vi "editDialog.vi"(0 "reference":refnum<class "ClassRelationshipEdge.lvclass">, 5 "error in (no error)":errorcluster) -> (14 "reference out":refnum<class "ClassRelationshipEdge.lvclass">, 15 "cancel":bool, 19 "error out":errorcluster)   [LabVIEW 2016, in "ClassRelationshipEdge.lvclass"]
doc: "Edit Dialog"
uses:
  <resource>/Framework/Providers/Open_GDS/UML/ClassRelationshipEdge_class/ClassRelationshipEdge.lvclass
  <resource>/Framework/Providers/Open_GDS/UML/ArrowHead_class/ArrowHeadType.ctl
  C:/Program Files (x86)/National Instruments/LabVIEW 2016/resource/Framework/Providers/Open_GDS/UML/SegmentedLineEdge_class/SegmentedLineEdge.lvclass
  <resource>/Framework/Providers/Open_GDS/UML/ContextHelp/ContextHelp_HelpTexts.ctl
  <resource>/Framework/Providers/Open_GDS/UML/ClassRelationshipEdge_class/private/AssociationType.ctl
  <resource>/Framework/Providers/Open_GDS/UML/BentStyle_class/BentStyle.lvclass
  <resource>/Framework/Providers/Open_GDS/UML/LineStyle_class/LineStyle.lvclass
  <resource>/Framework/Providers/Open_GDS/UML/ArrowHead_class/ArrowHead.lvclass
  <resource>/Framework/Providers/Open_GDS/UML/SegmentedLineEdge_class/SegmentedLineEdge.lvclass
panel:
  in  "SplitWire":bool
  in  "Bent Style 2":enum16{"STRAIGHT", "HV", "VH", "HVH", "VHV"}(ring) caption="bentStyle"
  in  "Help":bool
  in  "Bi directional":bool
  in  "Reverse association":bool
  in  "RelationType":u16(ring) items=["Dependency", "Inheritance", "Interface Implementation", "Association", "Aggregation", "Composite Aggregation"]
  in  "Line style":enum16{"SOLID", "DOTTED"}(ring)
  in  "Middle label":string(combo)
  in  "Start arrow head":T1
  in  "End arrow head":T1
  in  "Bent Style":enum16{"STRAIGHT", "HV", "VH", "HVH", "VHV"}(ring) caption="bentStyle"
  in  "Start label":string
  in  "End label":string
  in  "Cancel Button":bool
  in  "OK Button":bool
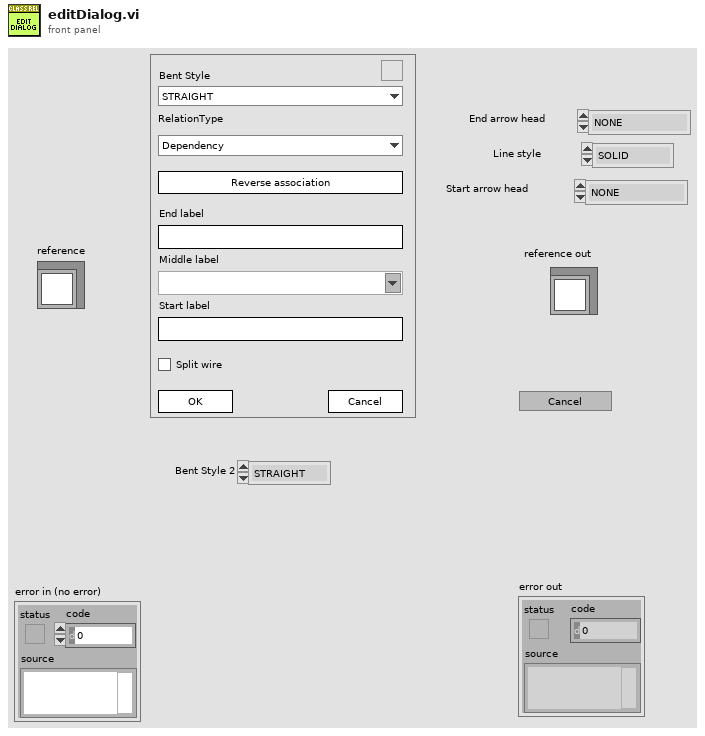
[diagram p1: front panel]
types:
  T1 = typedef "ArrowHead.lvclass/ArrowHeadType.ctl" = enum16{"NONE", "TRIANGLE", "BLACK_TRIANGLE", "V", "HALF_V", "DIAMOND", "BLACK_DIAMOND"}
  T2 = typedef "ContextHelp_HelpTexts.ctl" = enum16{"None(Hide)", "Default", "Help", "Welcome", "GettingStarted", "ClassDiagram_Help", "SequenceDiagram_Help", "UseCaseDiagram_Help", "BSelect", "BClass", "BInterface", "BPackage", "BNote", "BDependency", "BInheritance", "BInterfaceImplementation", "BAssociation", "BAggregation", "BCompAggregation", "BNoteConnector", "BObject", "BActionBar", "BCall", "BSystem", "BActor", "BUseCase", "BGeneralization", "BIncludes", "BExtends", "BUseCaseDiagramAssociation", "ClassRelationshipEdge editDialog_Bent Style", "ClassRelationshipEdge editDialog_RelationType", "ClassRelationshipEdge editDialog_Reverse association", "ClassRelationshipEdge editDialog_Start label", "ClassRelationshipEdge editDialog_Middle label", "ClassRelationshipEdge editDialog_End label", "UMLEditor reversedEngineering_Pathes", "ReversedEngineering StateReverseDialog_Help", "ReversedEngineering StateQueuedSettings_Help", "UMLEditor reversedEngineering_AddTopVIs", "UMLEditor reversedEngineering_AddClasses", "UMLEditor reversedEngineering_AddDirs", "UMLEditor reversedEngineering_Recursively", "UMLEditor reversedEngineering_Remove", "UMLEditor reversedEngineering_ClearList", "UMLEditor reversedEngineering_HideSubAss", "UMLEditor reversedEngineering_CreateTypes", "UMLEditor reversedEngineering_OnlyInheritance", "UMLEditor reversedEngineering_CreateApplication", "UMLEditor reversedEngineering_OK", "UMLEditor reversedEngineering_Cancel", "UMLEditor reversedEngineering_Help", "UMLEditor createWizardScriptFile_ScriptfilePath", "UMLEditor createWizardScriptFile_ClassPath", "UMLEditor createWizardScriptFile_Use", "UMLEditor createWizardScriptFile_PrivateDirName", "UMLEditor createWizardScriptFile_DirAppend", "UMLEditor createWizardScriptFile_Separator Character", "UMLEditor createWizardScriptFile_OK", "UMLEditor createWizardScriptFile_Cancel", "UMLEditor createWizardScriptFile_Help", "ClassNode editDialog_Class Name", "InterfaceNode editDialog_Class Name", "ClassNode editDialog_Attribute", "ClassNode editDialog_Methods", "InterfaceNode editDialog_Methods", "ClassNode editDialog_connection", "InterfaceNode editDialog_connection", "ClassNode editDialog_StereoType", "ClassNode editDialog_ShowAttrib", "ClassNode editDialog_ShowMethods", "ClassNode editDialog_ClassPath", "ClassNode editDialog_AddAttribute", "ClassNode editDialog_AddMethod", "InterfaceNode editDialog_AddMethod", "ClassNode AttributeGuide_AttributeName", "ClassNode AttributeGuide_Array?", "ClassNode AttributeGuide_Data Type", "ClassNode AttributeGuide_RefName", "ClassNode AttributeGuide_Preview", "ClassNode AttributeGuide_OK", "ClassNode AttributeGuide_Cancel", "ClassNode MethodGuide_Visibility", "ClassNode MethodGuide_Method Name", "ClassNode MethodGuide_Preview", "ClassNode MethodGuide_OK", "ClassNode MethodGuide_Cancel", "CallNode EditCallProperties_AllButtons", "ObjectNode EditObjectlProperties_AllButtons", "ActorNode EditActorProperties_AllButtons", "UseCaseRelationshipNode EditUseCaselProperties_AllButtons", "UseCaseNode EditUseCaselProperties_AllButtons", "SystemNode EditSystemProperties_AllButtons", "ReversedEngineering UpdateAttributes_AllButtons", "StateNode editDialog_AllButtons", "StateTransition editDialog_AllButtons", "ArrangeNodes Main_Picture", "ArrangeNodes Main_Zoom", "ArrangeNodes Main_Auto Zoom", "ArrangeNodes Main_shorten", "ArrangeNodes Main_Min Length", "ArrangeNodes Main_Max Length", "ArrangeNodes Main_increase", "ArrangeNodes Main_decrease", "ArrangeNodes Main_Shake", "ArrangeNodes Main", "BState", "BInitialState", "BFinalState", "BStateTransition", "StateDiagram_Help", "StateDiagram_PropertiesAllButtons", "ReversedEngineering StateReverseDialog_ClearStates", "ReversedEngineering StateReverseDialog_UseQueuedStateMachines", "ReversedEngineering StateReverseDialog_QueuedSettings", "ReversedEngineering StateReverseDialog_SearchForVIs", "ReversedEngineering StateReverseDialog_SearchCriteria", "OptionsDialog_ClassBasePath", "OptionsDialog_VIPath", "OptionsDialog_ApplicationPath", "OptionsDialog_WizDir", "OptionsDialog_IniFilePath", "OptionsDialog_DefineColors", "OptionsDialog_Help", "OptionsDialog_CreateTypes", "ClassRelationshipEdge editDialog_SplitWire"}
  T3 = typedef "ClassRelationshipEdge.lvclass/ObjectAttributes.ctl" = cluster{"bentStyleRef":refnum<class "BentStyle.lvclass">, "startConnectionOffset":cluster{"x":i32, "y":i32}, "endConnectionOffset":cluster{"x":i32, "y":i32}, "MidLineOffset":cluster{"x":i32, "y":i32}, "DepClass":T4}
  T4 = typedef "ReversedEngineering_ViDependencyDetailsType.ctl" = cluster{"ThisVIs/Ctls":path[], "Dependent_VIs/Ctls":path[]}
  T5 = typedef "SegmentedLineEdge.lvclass/ObjectAttributes.ctl" = cluster{"lineStyle":refnum<class "LineStyle.lvclass">, "startArrowHead":refnum<class "ArrowHead.lvclass">, "endArrowHead":refnum<class "ArrowHead.lvclass">, "startLabel":string, "midLabel":string, "endLabel":string, "MidLabelOffset":T6, "SplitWire":bool}
  T6 = typedef "Point Point2D.ctl" = cluster{"x":dbl, "y":dbl}
  T7 = typedef "ContextHelp_ShowType.ctl" = cluster{"Header":string, "Picture":picture, "Text":string}
  T8 = typedef "ClassRelationshipEdge.lvclass/AssociationType.ctl" = u16
  T9 = typedef "BentStyle.lvclass/BentStyleType.ctl" = enum16{"STRAIGHT", "HV", "VH", "HVH", "VHV", "ARC"}
  T10 = typedef "LineStyle.lvclass/LineStyleType.ctl" = enum16{"SOLID", "DOTTED"}
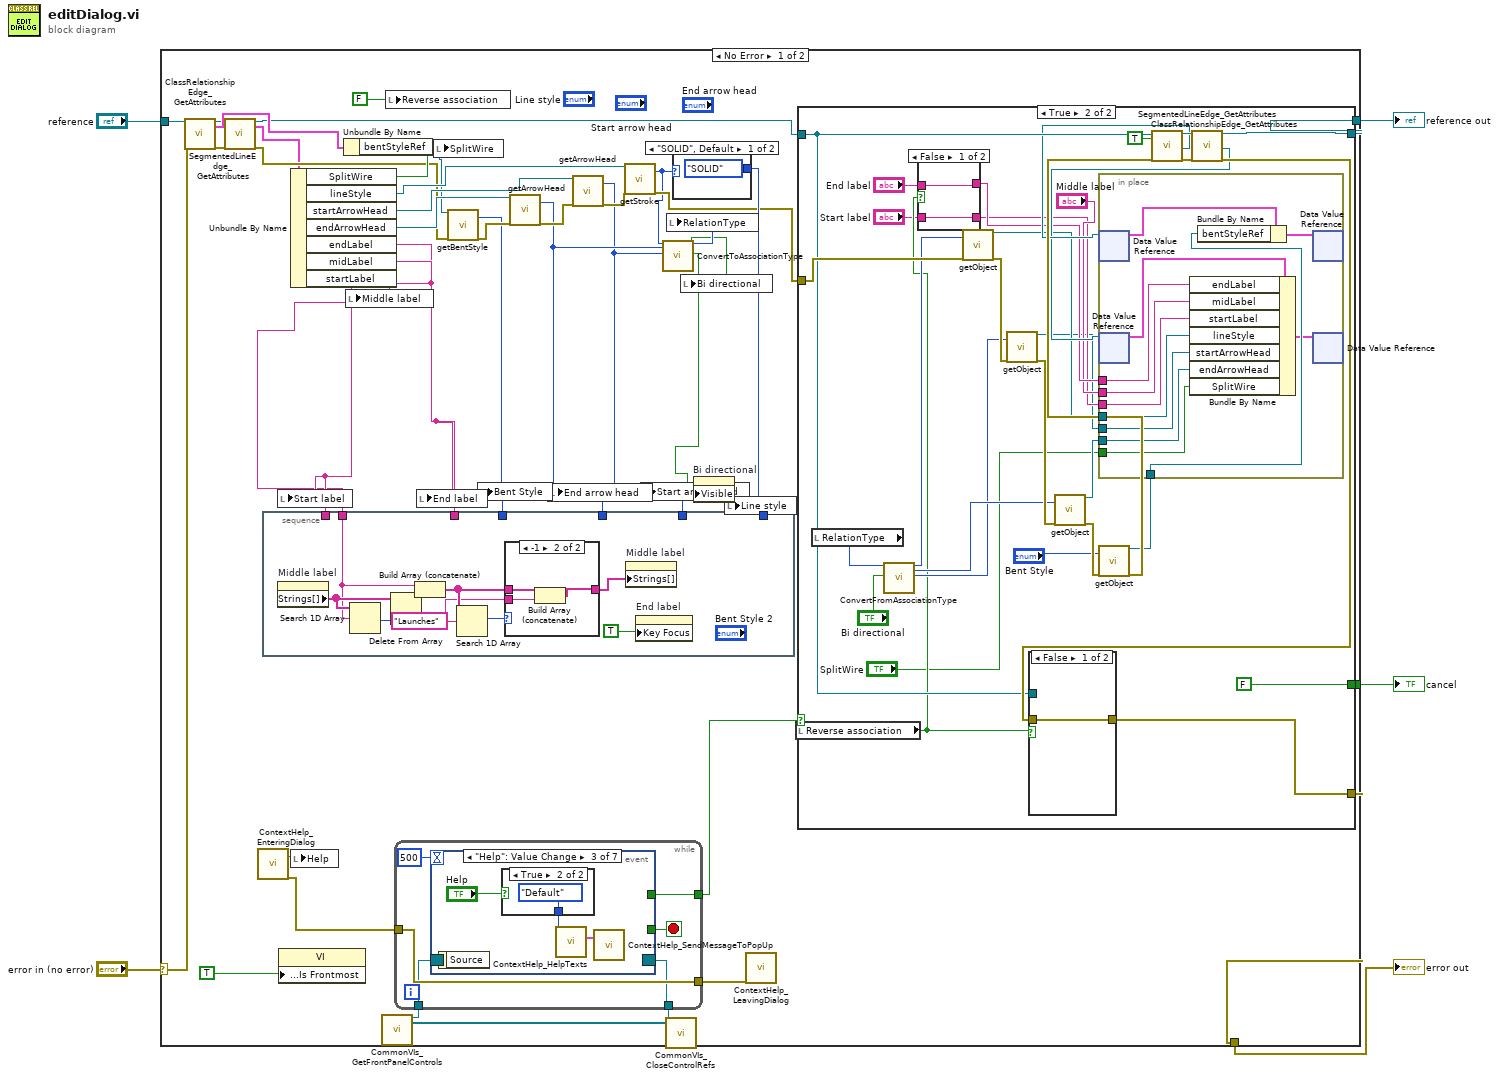
[diagram p0: block diagram]
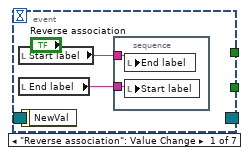
[diagram p2: hidden frame]
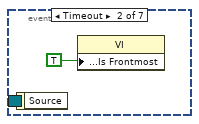
[diagram p3: hidden frame]
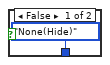
[diagram p4: hidden frame]
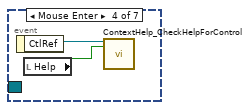
[diagram p5: hidden frame]
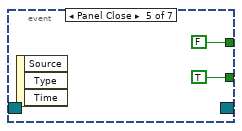
[diagram p6: hidden frame]
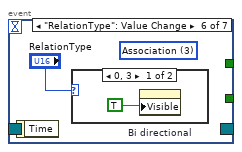
[diagram p7: hidden frame]
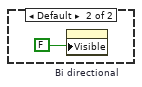
[diagram p8: hidden frame]
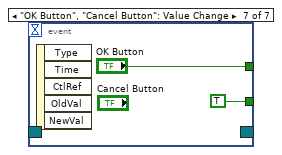
[diagram p9: hidden frame]
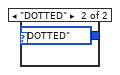
[diagram p10: hidden frame]
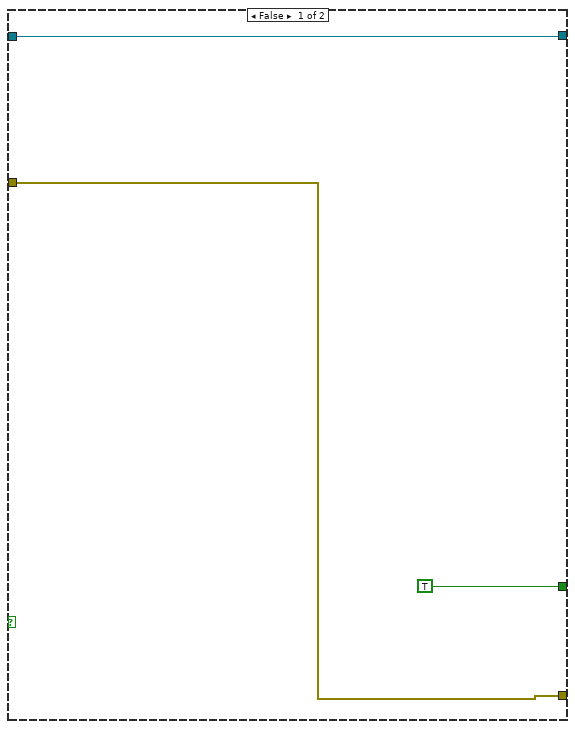
[diagram p11: hidden frame]
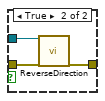
[diagram p13: hidden frame]
diagram:
  n1 = case shown="No Error" "error in (no error)" {
    selector: "error in (no error)" -> [w41 w140]
    tunnel: "reference" -> [w42 w141]
    tunnel: [w44 w140] -> w3
    tunnel: [w43 w141] -> w2
    tunnel: [w26 _] -> w1
    frame No Error {
      n2 = call <resource>:"ClassRelationshipEdge_GetAttributes.vi"("reference in"=w42, "error in (no error)"=w41) -> ("reference out"=w10:refnum<class "ClassRelationshipEdge.lvclass">, "Data"=w11:T3, "error out"=w9:errorcluster)  [unwired: 1 in, 14 out]
      n3 = call <resource>:"SegmentedLineEdge_GetAttributes.vi"("reference in"=w10, "error in (no error)"=w9) -> ("reference out"=w7:refnum<class "ClassRelationshipEdge.lvclass">, "Data"=w6:T5, "error out"=w8:errorcluster)  [unwired: 14 in, 1 out]
      n4 = call <resource>:"ContextHelp_EnteringDialog.vi"() -> ("HelpStatus"=w19:bool, "error out"=w18:errorcluster)  [unwired: 3 in, 15 out]
      n5 = property class="VI"("Front Panel Window:Is Frontmost"=TRUE) -> ()  [unwired: 2 in, 2 out]
      n6 = Unbundle By Name(w6) -> ("SplitWire"=w12:bool, "lineStyle"=w39:refnum<class "LineStyle.lvclass">, "startArrowHead"=w35:refnum<class "ArrowHead.lvclass">, "endArrowHead"=w33:refnum<class "ArrowHead.lvclass">, "endLabel"=w36:string, "midLabel"=w37:string, "startLabel"=w38:string)
      n7 = local write "Start label"(w38) -> ()
      n8 = local write "Help"(w19) -> ()
      n9 = Unbundle By Name(w11) -> ("bentStyleRef"=w30:refnum<class "BentStyle.lvclass">)
      n10 = local write "Middle label"(w37) -> ()
      n11 = call <resource>:"CommonVIs_GetFrontPanelControls.vi"() -> ("Event Registration Refnum"=w15:refnum<event-registration>, "ControlRefs"=w13:refnum<vi>[])  [unwired: 2 in, 16 out]
      n12 = local write "Reverse association"(FALSE ("Reverse association")) -> ()
      n13 = while {
        tunnel: [w50] -> w40
        tunnel: w18 -> [w48]
        tunnel: [w48] -> w17
        tunnel: w15 -> [w46]
        tunnel: [w45] -> w14
        stop <- w49 stop-if-true
        n14 = event shown="[2] \"Help\": Value Change" {
          selector: w46 -> [_ _ _ _ _ _ _]
          dyn-events: [_ _ _ _ _ _ _] -> w45
          timeout: 500 -> [_ _ _ _ _ _ _]
          tunnel: [_ _ _ _ FALSE ("OK Button") _ "OK Button"] -> w50
          tunnel: [_ _ _ _ TRUE _ TRUE] -> w49
          event "Reverse association": Value Change {
            n15 = local read "Start label"() -> (w52:string)
            n16 = local read "End label"() -> (w51:string)
            n17 = event-data() -> ()  [unwired: 2 out]
            n18 = stacked-sequence {
              tunnel: w52 -> [w54]
              tunnel: w51 -> [w53]
              frame #0 {
                n19 = local write "End label"(w54) -> ()
                n20 = local write "Start label"(w53) -> ()
              }
            }
          }
          event Timeout {
            n21 = event-data() -> ()  [unwired: 2 out]
            n22 = property class="VI"("Front Panel Window:Is Frontmost"=TRUE) -> ()  [unwired: 2 in, 2 out]
          }
          event "Help": Value Change {
            n23 = event-data() -> ()  [unwired: 2 out]
            n24 = case shown="True" "Help" {
              tunnel: [ContextHelp_HelpTexts."None(Hide)" ("HelpText") ContextHelp_HelpTexts."Default" ("HelpText")] -> w57
              frame False {
              }
              frame True {
              }
            }
            n25 = call <resource>:"ContextHelp_HelpTexts.vi"("HelpText (enum or string)"=w57) -> ("HelpOut"=w58:T7)  [unwired: 18 out]
            n26 = call <resource>:"ContextHelp_SendMessageToPopUp.vi"("PopUpMessage"=w58) -> ()  [unwired: 2 in, 17 out]
          }
          event Mouse Enter {
            n27 = event-data() -> ("CtlRef"=w62:refnum<vi>)  [unwired: 1 out]
            n28 = local read "Help"() -> (w61:bool)
            n29 = call <resource>:"ContextHelp_CheckHelpForControl.vi"("Ctl Refnum"=w62, "Help"=w61) -> ()  [unwired: 1 in, 17 out]
          }
          event Panel Close {
            n30 = event-data() -> ()  [unwired: 4 out]
          }
          event "RelationType": Value Change {
            (unwired) T8 3 items=["Depenency", "Inheritance", "Interface Implementation", "Association", "Aggregation", "Composite Aggregation"] ("RelationType")
            n31 = event-data() -> ()  [unwired: 2 out]
            n32 = case shown="0, 3" "RelationType" {
              frame 0, 3 {
                n33 = property on="Bi directional" class="Bool (strict)"("Visible"=TRUE) -> ()  [unwired: 2 in, 2 out]
              }
              frame Default {
                n34 = property on="Bi directional" class="Bool (strict)"("Visible"=FALSE) -> ()  [unwired: 2 in, 2 out]
              }
            }
          }
          event "OK Button", "Cancel Button": Value Change {
            n35 = event-data() -> ()  [unwired: 6 out]
          }
        }
      }
      n36 = local write "End label"(w36) -> ()
      n37 = local write "SplitWire"(w12) -> ()
      n38 = call-dynamic "getBentStyle.vi"("reference"=w30, "error in (no error)"=w8) -> ("bentStyle"=w27:T9, "error out"=w29:errorcluster)  [unwired: 15 in, 1 out]
      n39 = local write "Bent Style"(w27) -> ()
      n40 = call <resource>:"getArrowHead.vi"("reference"=w33, "error in (no error)"=w29) -> ("arrowHead"=w24:T1, "error out"=w32:errorcluster)  [unwired: 16 out]
      n41 = local write "End arrow head"(w24) -> ()
      n42 = call <resource>:"getArrowHead.vi"("reference"=w35, "error in (no error)"=w32) -> ("arrowHead"=w23:T1, "error out"=w31:errorcluster)  [unwired: 16 out]
      n43 = call-dynamic "getStroke.vi"("reference"=w39, "error in (no error)"=w31) -> ("lineStyle"=w25:T10, "error out"=w28:errorcluster)  [unwired: 15 in, 1 out]
      n44 = local write "Start arrow head"(w23) -> ()
      n45 = call <resource>:"ConvertToAssociationType.vi"("lineStyle"=w25, "EndArrowHead"=w24, "StartArrowHead"=w23) -> ("RelationType"=w22:T8, "Bi sirectional"=w21:bool)  [unwired: 15 out]
      n46 = call <resource>:"CommonVIs_CloseControlRefs.vi"("Event Registration Refnum"=w14, "ControlRefs"=w13) -> ()  [unwired: 1 in, 17 out]
      n47 = local write "RelationType"(w22) -> ()
      n48 = case shown="\"SOLID\", Default" w25 {
        tunnel: [enum16{"SOLID", "DOTTED"}."SOLID" ("Line style") enum16{"SOLID", "DOTTED"}."DOTTED" ("Line style")] -> w34
        frame "SOLID", Default {
        }
        frame "DOTTED" {
        }
      }
      n49 = stacked-sequence {
        tunnel: w34 -> [_]
        tunnel: w38 -> [_]
        tunnel: w37 -> [w132]
        tunnel: w36 -> [_]
        tunnel: w23 -> [_]
        tunnel: w24 -> [_]
        tunnel: w27 -> [_]
        frame #0 {
          w127 = "Launches" ("element")
          n50 = property on="Middle label" class="CmbBox"() -> ("Strings[]"=w134:string[])  [unwired: 2 in, 2 out]
          n51 = Search 1D Array(1D array=w134, element=w132) -> (index of element=w133:i32)  [unwired: 1 in]
          n52 = Delete From Array(array=w134, index=w133) -> (array with subset deleted=w131:string[])  [unwired: 1 in, 1 out]
          n53 = Build Array (concatenate)(w132, w131) -> (w129:string[])
          n54 = Search 1D Array(1D array=w129, element=w127) -> (index of element=w130:i32)  [unwired: 1 in]
          n55 = case shown="-1" w130 {
            tunnel: w129 -> [w136 w139]
            tunnel: [w136 w137] -> w128
            tunnel: w127 -> [_ w138]
            frame 0, Default {
            }
            frame -1 {
              n56 = Build Array (concatenate)(w139, w138) -> (w137:string[])
            }
          }
          n57 = property on="Middle label" class="CmbBox"("Strings[]"=w128) -> ()  [unwired: 2 in, 2 out]
          n58 = property on="End label" class="Str"("Key Focus"=TRUE) -> ()  [unwired: 2 in, 2 out]
        }
      }
      n59 = local write "Bi directional"(w21) -> ()
      n60 = property on="Bi directional" class="Bool (strict)"("Visible"=w21) -> ()  [unwired: 2 in, 2 out]
      n61 = local write "Line style"(w34) -> ()
      n62 = call <resource>:"ContextHelp_LeavingDialog.vi"("error in (no error)"=w17) -> ()  [unwired: 2 in, 17 out]
      n63 = case shown="True" w40 {
        tunnel: [w73 w93] -> w44
        tunnel: [w74 w106] -> w43
        tunnel: w7 -> [w74 w91]
        tunnel: w28 -> [w73 w101]
        tunnel: [TRUE ("Key Focus") FALSE ("Key Focus")] -> w26
        frame False {
        }
        frame True {
          n64 = local read "Reverse association"() -> (w90:bool)
          n65 = local read "RelationType"() -> (w97:u16)
          n66 = call <resource>:"ConvertFromAssociationType.vi"("RelationType"=w97, "Bi sirectional"="Bi directional") -> ("lineStyle"=w98:T10, "EndArrowHead"=w96:T1, "StartArrowHead"=w95:T1)  [unwired: 15 out]
          n67 = case shown="False" w90 {
            tunnel: "End label" -> [w120 w122]
            tunnel: [w119 w122] -> w79
            tunnel: [w120 w121] -> w81
            tunnel: "Start label" -> [w119 w121]
            frame False {
            }
            frame True {
            }
          }
          n68 = call <resource>:"getObject.vi"("lineStyle"=w98, "error in (no error)"=w101) -> ("reference out"=w78:refnum<class "LineStyle.lvclass">, "error out"=w105:errorcluster)  [unwired: 16 out]
          n69 = call <resource>:"getObject.vi"("arrowHead"=w95, "error in (no error)"=w105) -> ("reference out"=w77:refnum<class "ArrowHead.lvclass">, "error out"=w104:errorcluster)  [unwired: 16 out]
          n70 = call <resource>:"getObject.vi"("arrowHead"=w96, "error in (no error)"=w104) -> ("reference out"=w76:refnum<class "ArrowHead.lvclass">, "error out"=w103:errorcluster)  [unwired: 16 out]
          n71 = call <resource>:"getObject.vi"("bentStyle"="Bent Style", "error in (no error)"=w103) -> ("reference out"=w82:refnum<class "BentStyle.lvclass">, "error out"=w102:errorcluster)  [unwired: 16 out]
          n72 = call <resource>:"ClassRelationshipEdge_GetAttributes.vi"("reference in"=w91, "OnlyGetDvrReference(False)"=TRUE, "error in (no error)"=w102) -> ("reference out"=w86:refnum<class "ClassRelationshipEdge.lvclass">, "DataRef"=w84:refnum<data-value>, "error out"=w85:errorcluster)  [unwired: 13 in, 1 out]
          n73 = call <resource>:"SegmentedLineEdge_GetAttributes.vi"("reference in"=w86, "error in (no error)"=w85) -> ("reference out"=w106:refnum<class "ClassRelationshipEdge.lvclass">, "DataRef"=w83:refnum<data-value>, "error out"=w94:errorcluster)  [unwired: 14 in, 1 out]
          n74 = case shown="False" w90 {
            tunnel: w94 -> [w123 w126]
            tunnel: [w123 w125] -> w93
            tunnel: w91 -> [_ w124]
            frame False {
            }
            frame True {
              n75 = call-dynamic "ReverseDirection.vi"("reference"=w124, "error in (no error)"=w126) -> ("error out"=w125:errorcluster)  [unwired: 16 in, 1 out]
            }
          }
          n76 = in-place {
            in-place-border: w82 -> [w117]
            in-place-border: w81 -> [w114]
            in-place-border: "Middle label" -> [w113]
            in-place-border: w79 -> [w112]
            in-place-border: w78 -> [w111]
            in-place-border: w77 -> [w110]
            in-place-border: w76 -> [w109]
            in-place-border: "SplitWire" -> [w108]
            n77 = in-place-dvr #1(w84) -> (w118:T3)  [unwired: 1 out]
            n78 = in-place-dvr #2(w83) -> (w115:T5)  [unwired: 1 out]
            n79 = Bundle By Name(cluster=w115, "endLabel"=w114, "midLabel"=w113, "startLabel"=w112, "lineStyle"=w111, "startArrowHead"=w110, "endArrowHead"=w109, "SplitWire"=w108) -> (w107:T5)
            n80 = Bundle By Name(cluster=w118, "bentStyleRef"=w117) -> (w116:T3)
            n81 = in-place-dvr #1(w116) -> ()  [unwired: 2 out]
            n82 = in-place-dvr #2(w107) -> ()  [unwired: 2 out]
          }
        }
      }
    }
    frame Error {
    }
  }
  "reference out" <- w2
  "error out" <- w3
  "cancel" <- w1
